vi "Read Cluster Data.vi"(7 "Section Name":string, 8 "error in (no error)":errorcluster, 10 "Clust Refnum":refnum<vi>, 11 "File Refnum":T1) -> (0 "error out":errorcluster, 3 "dup Clust Refnum":refnum<vi>)   [LabVIEW 2021, in "CANOpen Addon System Explorer.lvlib"]
uses:
  CANOpen Addon System Explorer.lvlib
  <vilib>/Utility/config.llb/Config Data RefNum.ctl
  <vilib>/Utility/config.llb/NI_LVConfig.lvlib
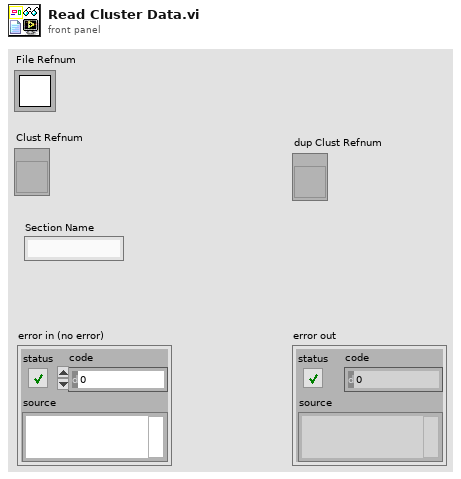
[diagram p1: front panel]
types:
  T1 = typedef "NI_LVConfig.lvlib/Config Data RefNum.ctl" = refnum<k1>
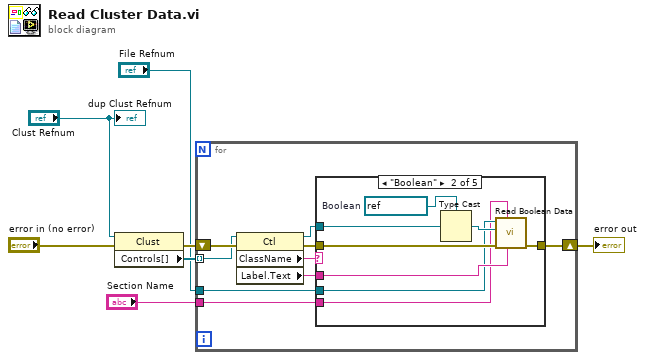
[diagram p0: block diagram]
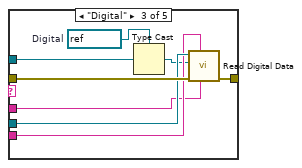
[diagram p3: hidden frame]
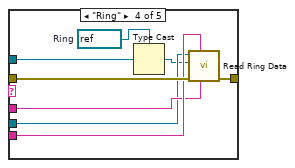
[diagram p4: hidden frame]
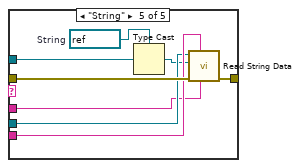
[diagram p5: hidden frame]
diagram:
  n1 = property class="Clust"(reference="Clust Refnum", error in="error in (no error)") -> (error out=w5:errorcluster, "Controls[]"=w6:refnum<vi>[])  [unwired: 1 out]
  n2 = for {
    tunnel: w6 -> [w8] mode=indexing
    shift-right: [w14] -> w3
    shift-left: w5 -> [w9]
    tunnel: "Section Name" -> [w16]
    tunnel: "File Refnum" -> [w15]
    n3 = property class="Ctl"(reference=w8, error in=w9) -> (reference out=w11:refnum<vi>, error out=w12:errorcluster, "ClassName"=w13:string, "Label.Text"=w10:string)
    n4 = case shown="\"Boolean\"" w13 {
      tunnel: w16 -> [_ w18 w31 w39 w47]
      tunnel: w15 -> [_ w20 w32 w37 w46]
      tunnel: w12 -> [w17 w23 w33 w40 w49]
      tunnel: w11 -> [_ w19 w28 w36 w45]
      tunnel: [w17 w21 w30 w41 w48] -> w14
      tunnel: w10 -> [_ w22 w29 w38 w42]
      frame "others", Default {
      }
      frame "Boolean" {
        w24 = refnum<vi> refnum  # Boolean
        n5 = Type Cast(type=w24, x=w19) -> (*(type *) &x=w25:refnum<vi>)
        n6 = call "Read Boolean Data.vi"("Keyword Name"=w22, "Section Name"=w18, "error in (no error)"=w23, "Bool Refnum"=w25, "File Refnum"=w20) -> ("error out"=w21:errorcluster)  [unwired: 6 in]
      }
      frame "Digital" {
        w26 = refnum<vi> refnum  # Digital
        n7 = Type Cast(type=w26, x=w28) -> (*(type *) &x=w27:refnum<vi>)
        n8 = call "Read Digital Data.vi"("Keyword Name"=w29, "Section Name"=w31, "error in (no error)"=w33, "DigNum Refnum"=w27, "file refnum"=w32) -> ("error out"=w30:errorcluster)  [unwired: 6 in]
      }
      frame "Ring" {
        w34 = refnum<vi> refnum  # Ring
        n9 = Type Cast(type=w34, x=w36) -> (*(type *) &x=w35:refnum<vi>)
        n10 = call "Read Ring Data.vi"("Keyword Name"=w38, "Section Name"=w39, "error in (no error)"=w40, "Ring Refnum"=w35, "File Refnum"=w37) -> ("error out"=w41:errorcluster)  [unwired: 6 in]
      }
      frame "String" {
        w44 = refnum<vi> refnum  # String
        n11 = Type Cast(type=w44, x=w45) -> (*(type *) &x=w43:refnum<vi>)
        n12 = call "Read String Data.vi"("Keyword Name"=w42, "Section Name"=w47, "error in (no error)"=w49, "Str Refnum"=w43, "File Refnum"=w46) -> ("error out"=w48:errorcluster)  [unwired: 6 in]
      }
    }
  }
  "error out" <- w3
  "dup Clust Refnum" <- "Clust Refnum"
